vi "GetFOV.vi"(4 "connection ID in":refnum<k5>, 5 "Timeout (ms)":i32=40000000) -> (0 "Roi Lat Min":dbl format="%.2f", 1 "connection ID out":refnum<k5>, 2 "Roi Lat Span":dbl format="%.2f")   [LabVIEW 2016]
uses:
  TemperatureMeasure/Thermal_type.vi
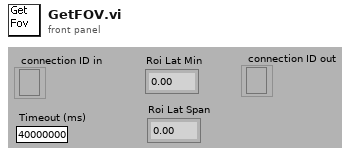
[diagram p1: front panel]
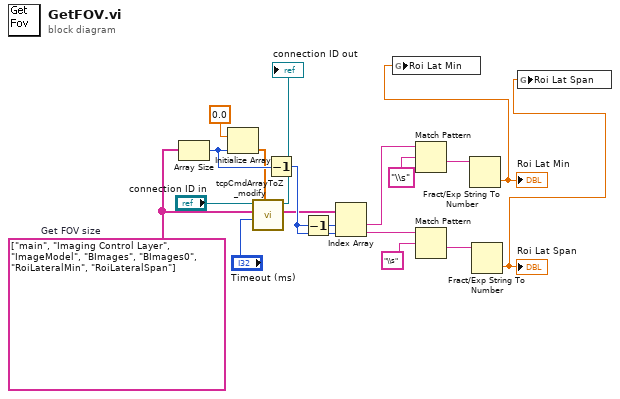
[diagram p0: block diagram]
diagram:
  w15 = string[] ["main", "Imaging Control Layer", "ImageModel", "BImages", "BImages0", "RoiLateralMin", "RoiLateralSpan"]  # Get FOV size
  n1 = Array Size(array=w15) -> (size(s)=w17:i32)
  n2 = Initialize Array(0.0 ("delay (sec)"), w17) -> (w16:dbl[])
  n3 = call "tcpCmdArrayToZ_modify.vi"("Delay (sec)"=w16, "Timeout (ms)"="Timeout (ms)", "Command array"=w15, "connection ID in"="connection ID in") -> ("Receive array"=w8:string[], "connection ID out"=→"connection ID out":refnum<k5>)  [unwired: 3 in, 3 out]
  n4 = Decrement(x=w17) -> (x-1=w14:i32)
  n5 = Decrement(x=w14) -> (x-1=w13:i32)
  n6 = Index Array(array=w8, index #1=w13, index #2=w14) -> (element #1=w10:string, element #2=w11:string)
  n7 = Match Pattern(string=w10, regular expression="\\s" ("match pattern")) -> (after substring=w7:string)  [unwired: 1 in, 3 out]
  n8 = Match Pattern(string=w11, regular expression="\\s" ("match pattern")) -> (after substring=w6:string)  [unwired: 1 in, 3 out]
  n9 = Fract/Exp String To Number(string=w7) -> (number=w2:dbl)  [unwired: 3 in, 1 out]
  "Roi Lat Min" <- w2
  n10 = global write "Thermal_type.vi" "Roi Lat Min"(w2) -> ()
  n11 = Fract/Exp String To Number(string=w6) -> (number=w3:dbl)  [unwired: 3 in, 1 out]
  "Roi Lat Span" <- w3
  n12 = global write "Thermal_type.vi" "Roi Lat Span"(w3) -> ()
